vi "to string array.vi"(8 "error in (no error)":errorcluster, 11 "module configuration in":refnum<class "Modbus Module configuration.lvclass">) -> (0 "error out":errorcluster, 1 "Array":string[][](array[string]), 2 "version":string, 3 "module configuration out":refnum<class "Modbus Module configuration.lvclass">)   [LabVIEW 2015, in "Modbus Module configuration.lvclass"]
uses:
  Modbus Module configuration.lvclass
  Modbus Module configuration.lvclass/Modbus Module configuration.ctl
  <vilib>/NI/Tag Bus/tag/tag descriptor.lvclass/tag descriptor.ctl
  <vilib>/NI/Tag Bus Module Framework/channel/TBM channel.lvclass/TBM channel.ctl
  <vilib>/NI/Tag Bus/tag/read tag name.vi
  <vilib>/NI/Tag Bus Module Framework/channel/Read channel classification.vi
  <vilib>/NI/Tag Bus/tag/read data type.vi
  editor node/Modbus Module editor node.lvclass
  module channel/Modbus Module Channel.lvclass
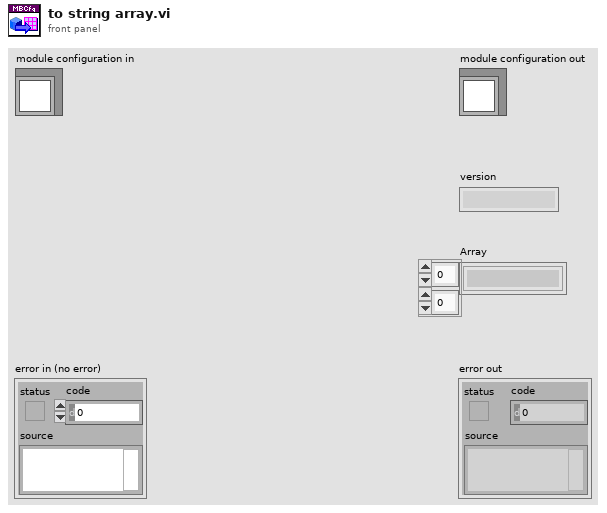
[diagram p1: front panel]
types:
  T1 = typedef "TBM channel.lvclass/channel classification.ctl" = enum16{"input data", "output data", "processing parameter", "processing result"}
  T2 = typedef "tag bus.lvlib/tag descriptor.lvclass/Data Type.ctl" = enum16{"Double", "Single", "I64", "I32", "I16", "I8", "U64", "U32", "U16", "U8", "Boolean", "String", "Array of Double", "Array of Single", "Array of I64", "Array of I32", "Array of I16", "Array of I8", "Array of U64", "Array of U32", "Array of U16", "Array of U8", "Array of Boolean", "Array of String"}
  T3 = typedef "Modbus Module editor node.lvclass/permissions.ctl" = enum32{"Read from MB", "Write to MB"}
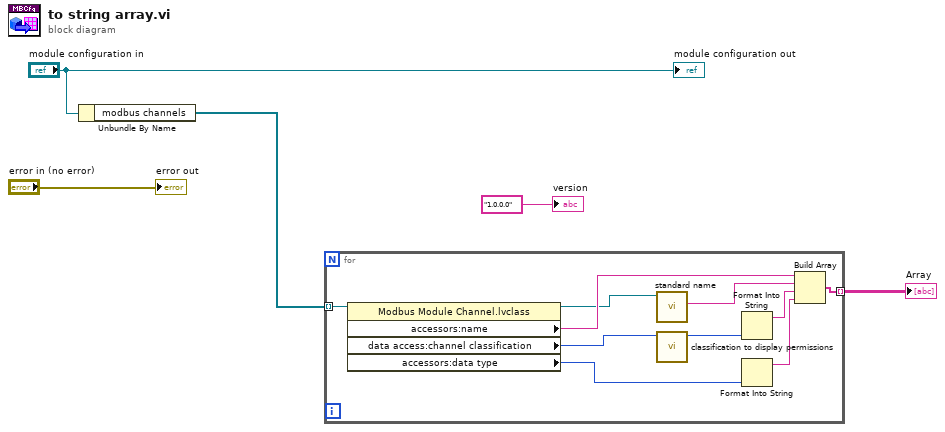
[diagram p0: block diagram]
diagram:
  n1 = Unbundle By Name("module configuration in") -> ("modbus channels"=w2:refnum<class "Modbus Module Channel.lvclass">[])
  n2 = for {
    tunnel: w2 -> [w8] mode=indexing
    tunnel: [w7] -> w1 mode=indexing
    n3 = property class="Modbus Module Channel.lvclass"(reference=w8) -> (reference out=w9:refnum<class "Modbus Module Channel.lvclass">, "accessors:name"=w11:string, "data access:channel classification"=w12:T1, "accessors:data type"=w10:T2)  [unwired: 1 in, 1 out]
    n4 = call "standard name.vi"("Modbus Module Channel in"=w9) -> ("standard name"=w6:string)  [unwired: 8 in, 2 out]
    n5 = call "classification to display permissions.vi"("channel classification"=w12) -> ("permissions"=w14:T3)  [unwired: 10 in]
    n6 = Format Into String(w14) -> (resulting string=w13:string)  [unwired: 3 in, 1 out]
    n7 = Format Into String(w10) -> (resulting string=w15:string)  [unwired: 3 in, 1 out]
    n8 = Build Array(w11, w6, w13, w15) -> (w7:string[])
  }
  "Array" <- w1
  "error out" <- "error in (no error)"
  "module configuration out" <- "module configuration in"
  "version" <- "1.0.0.0" ("version")
